vi "Inspect Fiducials.vi"(7 "Console Log in":refnum<class "Console Log.lvclass">, 8 "error in":errorcluster, 11 "Potting Procedure in":refnum<class "Potting Procedure.lvclass">) -> (0 "error out":errorcluster, 3 "Potting Procedure out":refnum<class "Potting Procedure.lvclass">, 5 "Console Log out":refnum<class "Console Log.lvclass">)   [LabVIEW 2011, in "Potting Procedure.lvclass"]
uses:
  Potting Procedure.lvclass
  UI Classes/Console Log/Console Log.lvclass
  Shared Components/Utils/Type Definitions/Fiducial Image.ctl
  Shared Components/Utils/Type Definitions/Physical Image.ctl
  Shared Components/Vec3d Class/Vec3d Class.lvclass
  <vilib>/vision/Image Controls.llb/IMAQ Image.ctl
  Shared Components/Utils/Type Definitions/Fiducial with Source.ctl
  Type Definitions/Inspect Fiducials.ctl
  Potting Procedure.lvclass/Potting Procedure.ctl
  Shared Components/Gantry Class/Gantry Class.lvclass
  Shared Components/CameraTool Class/CameraTool Class.lvclass
  Shared Components/WorkTable Class/WorkTable Class.lvclass
  Shared Components/Config Manager Class/Type Definitions/Part Type.ctl
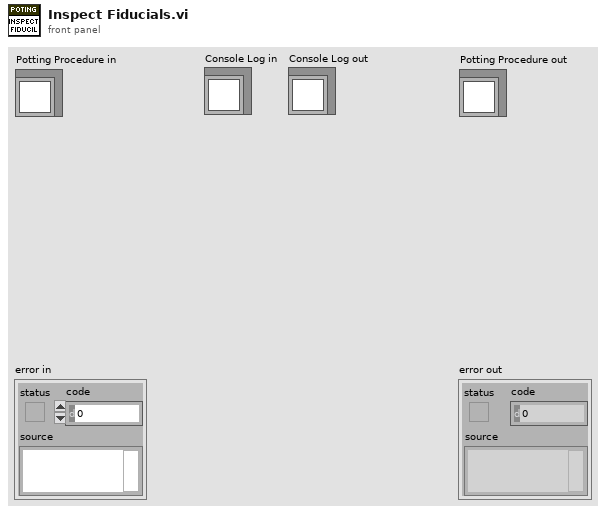
[diagram p1: front panel]
types:
  T1 = typedef "Fiducial Image.ctl" = cluster{"Fiducial Image":T2, "Selected Fiducial":T4, "fiducial name":string}
  T2 = typedef "Physical Image.ctl" = cluster{"Image Position":refnum<class "Vec3d Class.lvclass">, "Image Reference":T3, "Field of View":cluster{"x(mm)":dbl, "y(mm)":dbl}}
  T3 = typedef "IMAQ Image.ctl" = refnum<image>
  T4 = typedef "Fiducial with Source.ctl" = cluster{"Fiducial Image Coordinate":refnum<class "Vec3d Class.lvclass">, "Fiducial Source":enum16{"Pattern Recognition", "User", "Error", "Default"}}
  T5 = cluster{"Fiducials-HDI":T1[], "Fiducials-BBM":T1[], "Chuck":i32, "Slot":i32}[]
  T6 = typedef "Inspect Fiducials.ctl" = cluster{"Has Been Run?":bool, "Module-Chuck Fiducials":cluster{"Fiducials-HDI":T1[], "Fiducials-BBM":T1[], "Chuck":i32, "Slot":i32}[]}
  T7 = enum16{"Empty", "Unglued", "Stamped", "PartOnTop", "Weighted", "Unpotted", "Potted"}
  T8 = typedef "Part Type.ctl" = enum16{"BBM", "HDI", "GLUERESERVOIR", "STAMP", "WEIGHT"}
  T9 = cluster{"Fiducials-HDI":T1[], "Fiducials-BBM":T1[], "Chuck":i32, "Slot":i32}
  T10 = typedef "Worktable_Module Slot.ctl" = cluster{"Slot State":enum16{"Empty", "Unglued", "Stamped", "PartOnTop", "Weighted", "Unpotted", "Potted"}, "BBM Type":enum16{"None", "BBM", "GlassSlide"}, "HDI Type":enum16{"None", "HDI", "Polyimide"}, "Vacuum Channel":u8, "Location/Orientation BBM":T11, "Location/Orientation HDI":T11, "S/N":string}
  T11 = typedef "Position_Orientation.ctl" = cluster{"Center":refnum<class "Vec3d Class.lvclass">, "Orientation":refnum<class "Orient3d Class.lvclass">}
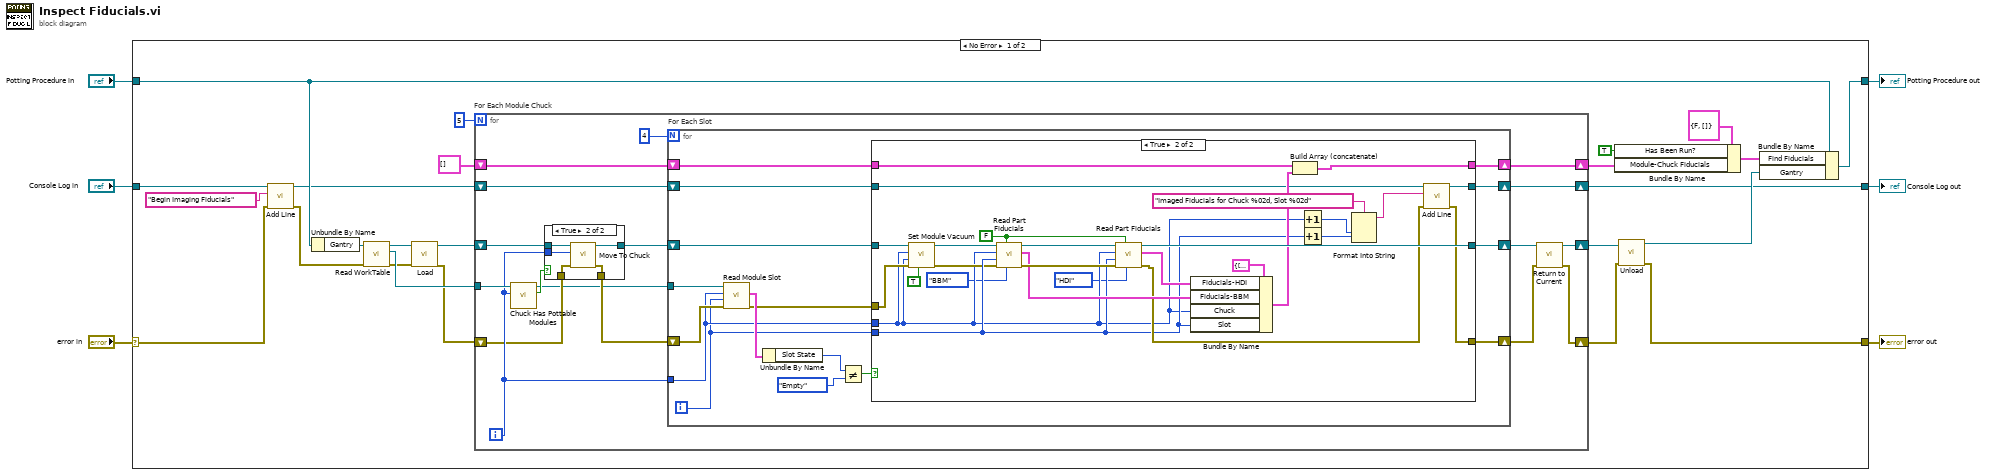
[diagram p0: block diagram]
diagram:
  n1 = case shown="No Error" "error in" {
    selector: "error in" -> [w10 w104]
    tunnel: [w19 w104] -> w5
    tunnel: [w18 w103] -> w3
    tunnel: "Potting Procedure in" -> [w21 w103]
    tunnel: "Console Log in" -> [w12 w102]
    tunnel: [w15 w102] -> w1
    frame No Error {
      n2 = call "Add Line.vi"("error in"=w10, "String"="Begin Imaging Fiducials", "Console Log in"=w12) -> ("error out"=w9:errorcluster, "Console Log out"=w11:refnum<class "Console Log.lvclass">)  [unwired: 7 in]
      n3 = Unbundle By Name(w21) -> ("Gantry"=w30:refnum<class "Gantry Class.lvclass">)
      n4 = call-dynamic "Read WorkTable.vi"("error in"=w9, "Gantry Class in"=w30) -> ("error out"=w8:errorcluster, "WorkTable Class.lvclass"=w28:refnum<class "WorkTable Class.lvclass">, "Gantry Class out"=w29:refnum<class "Gantry Class.lvclass">)  [unwired: 7 in]
      n5 = call "Load.vi"("error in"=w8, "Gantry In"=w29) -> ("error out"=w26:errorcluster, "CameraTool out"=w25:refnum<class "CameraTool Class.lvclass">)  [unwired: 8 in]
      n6 = for "For Each Module Chuck" {
        N: 5 -> [_]
        tunnel: w28 -> [w36]
        shift-right: [w39] -> w22
        shift-left: w25 -> [w42]
        shift-right: [w37] -> w20
        shift-left: w26 -> [w33]
        shift-right: [w45] -> w13
        shift-left: T5 [] ("Module-Chuck Fiducials") -> [w46]
        shift-right: [w43] -> w15
        shift-left: w11 -> [w44]
        i -> [w35]
        n7 = call "Chuck Has Pottable Modules.vi"("Chuck"=w35, "WorkTable in"=w36) -> ("Has Pottable Modules"=w34:bool, "WorkTable out"=w31:refnum<class "WorkTable Class.lvclass">)  [unwired: 7 in, 1 out]
        n8 = case shown="True" w34 {
          tunnel: w42 -> [w49 w54]
          tunnel: [w49 w53] -> w41
          tunnel: w35 -> [_ w52]
          tunnel: w33 -> [w48 w51]
          tunnel: [w48 w50] -> w32
          frame False {
          }
          frame True {
            n9 = call-dynamic "Move To Chuck.vi"("error in"=w51, "Chuck"=w52, "Gantry in"=w54) -> ("error out"=w50:errorcluster, "Gantry out"=w53:refnum<class "CameraTool Class.lvclass">)  [unwired: 7 in]
          }
        }
        n10 = for "For Each Slot" {
          N: 4 -> [_]
          tunnel: w35 -> [w64]
          shift-right: [w61] -> w40
          shift-left: w41 -> [w65]
          shift-right: [w60] -> w38
          shift-left: w32 -> [w70]
          shift-right: [w58] -> w45
          shift-left: w46 -> [w59]
          shift-right: [w56] -> w43
          shift-left: w44 -> [w57]
          tunnel: w31 -> [w55]
          i -> [w63]
          n11 = call-dynamic "Read Module Slot.vi"("error in"=w70, "slot"=w63, "chuck"=w64, "WorkTable in"=w55) -> ("error out"=w62:errorcluster, "Module Slot"=w69:T10)  [unwired: 5 in, 1 out]
          n12 = Unbundle By Name(w69) -> ("Slot State"=w67:T7)
          n13 = Not Equal?(x=w67, y=T7."Empty" ("BBM Slot State")) -> (x != y?=w66:bool)
          n14 = case shown="True" w66 {
            tunnel: w65 -> [w74 w82]
            tunnel: w64 -> [_ w78]
            tunnel: w63 -> [_ w84]
            tunnel: w62 -> [w73 w79]
            tunnel: [w74 w96] -> w61
            tunnel: [w73 w89] -> w60
            tunnel: w59 -> [w72 w95]
            tunnel: [w72 w93] -> w58
            tunnel: w57 -> [w71 w92]
            tunnel: [w71 w91] -> w56
            frame False {
            }
            frame True {
              w100 = FALSE ("Dispose Images?")
              n15 = call-dynamic "Set Module Vacuum.vi"("On/Off"=TRUE, "error in"=w79, "Slot Number"=w78, "Chuck Number"=w78, "Gantry in"=w82) -> ("error out"=w80:errorcluster, "Gantry out"=w81:refnum<class "CameraTool Class.lvclass">)  [unwired: 5 in]
              n16 = call-dynamic "Read Part Fiducials.vi"("Part Type"=Part_Type."BBM", "Dispose Images?"=w100, "error in"=w80, "Slot"=w84, "Chuck"=w78, "CameraTool in"=w81) -> ("error out"=w99:errorcluster, "Fiducials"=w97:T1[], "CameraTool out"=w101:refnum<class "CameraTool Class.lvclass">)  [unwired: 3 in]
              n17 = call-dynamic "Read Part Fiducials.vi"("Part Type"=Part_Type."HDI", "Dispose Images?"=w100, "error in"=w99, "Slot"=w84, "Chuck"=w78, "CameraTool in"=w101) -> ("error out"=w90:errorcluster, "Fiducials"=w98:T1[], "CameraTool out"=w96:refnum<class "CameraTool Class.lvclass">)  [unwired: 3 in]
              n18 = Bundle By Name(cluster=T9 {"Fiducials-HDI"=[], "Fiducials-BBM"=[], "Chuck"=0, "Slot"=0} ("Module Fiducials"), "Fiducials-HDI"=w98, "Fiducials-BBM"=w97, "Chuck"=w78, "Slot"=w84) -> (w94:T9)
              n19 = Build Array (concatenate)(w95, w94) -> (w93:T5)
              n20 = Increment(x=w78) -> (x+1=w86:i32)
              n21 = Increment(x=w84) -> (x+1=w85:i32)
              n22 = Format Into String(format string="Imaged Fiducials for Chuck %02d, Slot %02d", w86, w85) -> (resulting string=w88:string)  [unwired: 2 in, 1 out]
              n23 = call "Add Line.vi"("error in"=w90, "String"=w88, "Console Log in"=w92) -> ("error out"=w89:errorcluster, "Console Log out"=w91:refnum<class "Console Log.lvclass">)  [unwired: 7 in]
            }
          }
        }
        n24 = call-dynamic "Return to Current.vi"("error in"=w38, "Gantry in"=w40) -> ("error out"=w37:errorcluster, "Gantry out"=w39:refnum<class "CameraTool Class.lvclass">)  [unwired: 8 in]
      }
      n25 = Bundle By Name(cluster=T6 {"Has Been Run?"=FALSE, "Module-Chuck Fiducials"=[]} ("Find Fiducials"), "Has Been Run?"=TRUE, "Module-Chuck Fiducials"=w13) -> (w16:T6)
      n26 = call "Unload.vi"("error in"=w20, "CameraTool in"=w22) -> ("error out"=w19:errorcluster, "Gantry out"=w17:refnum<class "Gantry Class.lvclass">)  [unwired: 8 in]
      n27 = Bundle By Name(cluster=w21, "Find Fiducials"=w16, "Gantry"=w17) -> (w18:refnum<class "Potting Procedure.lvclass">)
    }
    frame Error {
    }
  }
  "error out" <- w5
  "Potting Procedure out" <- w3
  "Console Log out" <- w1
